vi "Set Encoder Mode [ENCM].vi"(7 "Micropulse # In":i32, 8 "error in (no error)":errorcluster, 10 "Encoder Mode":T1=enum."32-bit + LLC") -> (0 "error out":errorcluster, 5 "Micropulse # Out":i32)   [LabVIEW 2026, in "MicroPulse_Driver.lvlib"]
doc: "This command allows the global setting of encoder parameters. Mode 0 is the default mode of 24-bit encoders with the standard output message format. Mode 1 is the full 32-bit output mode. In mode 2 the output mode is full 32 bit but also the output message of inspection modes FLR and FLX/FLZ are now a 32-bit LLC message giving all axis positions instead of the normal LCI message that only gave information about a single axis. Further modes are available 3, 4, and 5 that give the same as modes 0, 1 and 2 but also include with the axis data a message that gives the status of the input/output lines. This message is the same as the reply to an STS 6 command.\n\nThe input mode and filter count are optional parameters. The input mode sets all axis as either full Quadrature or Step/Direction. In Step/Direction the ‘A+’ input is the Step whilst the ‘B+’ is the Direction. Each complete Step pulse is two encoder counts. The filter count is a parameter that can used to clean up the edges of noisy encoders by time hysteresis. This defines the length of time before a decision is made on any input transitions and can filter out noise spikes and noisy level transitions.\nFor individual setting of the Input Mode and Filter Count see the ENCT and ENCF command respectively. It is recommended that these are used.\n\nThe optional fourth parameter (LLC Freq) allows the setting of an increased number of LLC messages (as defined by the Mode parameter above). Normally only one LLC is sent at the start of a data set. If this parameter is used then an LLC will be still sent at the start of a data set, but then further LLC messages will be sent during the data set on before every nth test.\n\nParameters:\n<Mode> : Integer value from 0 to 5:\n0 = 24 Bit output (Default)\n1 = 32 Bit output\n2 = 32 Bit output with LLC message for moving inspection modes\n3 = 24 Bit output with STS 6 message\n4 = 32 Bit output with STS 6 message\n5 = 32 Bit output with LLC message for moving inspection modes with STS 6 message\n\n[Input Mode] : Integer 0 or 1:\n0 = Quadrature (Default)\n1 = Step/Direction\n\n[Filter Count] : Integer value from 0 to 255:\n0 = OFF (Default 0)\n1 to 255 = approximately 100nSec to 20uSec\n\n[LLC Freq] : Integer value \"n\" from 0 to 100 (default 0).\n\nNote:\nThe 32-bit encoders require longer messages for LLC, LCI and LCA. The format is shown in the MicroPulse Output Messages Section.\n\nSystem Compatibility:\nLT1 supports only mode 0 – 2"
uses:
  MicroPulse_Driver.lvlib
  Data/Datatypes/MP - encoder mode.ctl
  Private/MP-Registry Action-Enum.ctl
  <instrlib>/Micropulse/Micropulse.lvlib
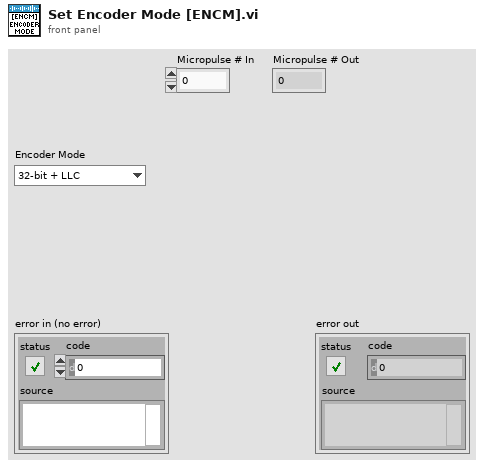
[diagram p1: front panel]
types:
  T1 = typedef "Micropulse.lvlib/MP - encoder mode.ctl" = enum16{"24-bit + LCI", "32-bit + LCI", "32-bit + LLC", "24-bit + STS6", "32-bit + STS6", "32-bit + LLC+STS6"}
  T2 = typedef "MicroPulse_Driver.lvlib/MP-Registry Action-Enum.ctl" = enum16{"Read", "Add Test", "Add Command", "Add Gate Command", "Add Encoder Command", "Clear Command  List", "Set Registry", "Set System Details", "Set DOF", "Set Velocity", "Disable Asynch Reads", "Enable Asynch Reads", "Add Connection", "Disconnect", "Shutdown"}
  T3 = typedef "Micropulse.lvlib/TCP config.ctl" = cluster{"Connection ID":refnum<k5>, "IP address":string, "host port":u16, "OC timeout":i32, "Read timeout":i32, "Write timeout":i32}
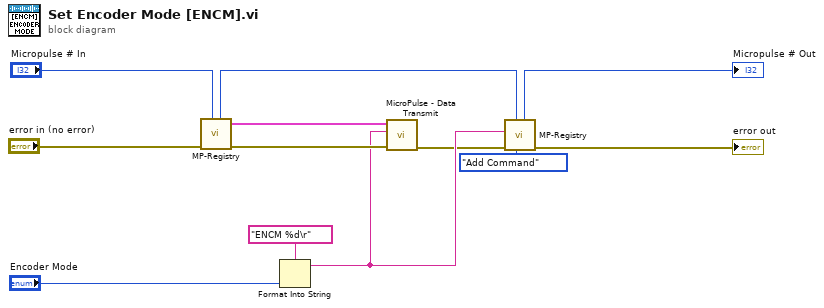
[diagram p0: block diagram]
diagram:
  n1 = call "MP-Registry.vi"("Micropulse # In"="Micropulse # In", "error in (no error)"="error in (no error)") -> ("error out"=w10:errorcluster, "TCP config"=w9:T3, "Micropulse # Out"=w5:i32)  [unwired: 6 in, 1 out]
  n2 = Format Into String(format string="ENCM %d\r", "Encoder Mode") -> (resulting string=w8:string)  [unwired: 2 in, 1 out]
  n3 = call "MicroPulse - Data Transmit.vi"("error in (no error)"=w10, "data"=w8, "TCP config"=w9) -> ("error out"=w6:errorcluster)  [unwired: 6 in, 2 out]
  n4 = call "MP-Registry.vi"("Action"=MP-Registry_Action-Enum."Add Command", "Micropulse # In"=w5, "error in (no error)"=w6, "Data in"=w8) -> ("error out"=→"error out":errorcluster, "Micropulse # Out"=→"Micropulse # Out":i32)  [unwired: 4 in, 2 out]
